vi "PT DIM info service.vi"(1 "serviceName":string, 3 "timeout [ms]":u32=10000, 5 "error in (no error)":errorcluster) -> (14 "serviceID":u32, 15 "data":i8[](array[numeric]), 16 "typeDescriptor":string, 17 "timed out?":bool, 19 "error out":errorcluster)   [LabVIEW 2014, in "PTUtils.lvlib"]
uses:
  PTUtils.lvlib
  CSlibraries-extern/DimLVEvent/LVDimInterface/LVDimInterface.dim service type.ctl
  CSlibraries-extern/DimLVEvent/LVDimInterface/LVDimInterface.dic_info_service_notifier.vi
  CSlibraries-extern/DimLVEvent/LVDimInterface/LVDimInterface.lvlib
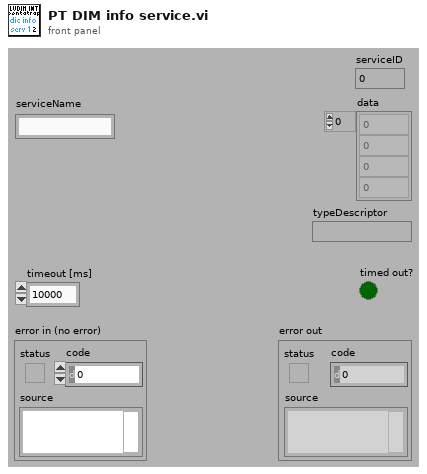
[diagram p1: front panel]
types:
  T1 = typedef "LVDimInterface.lvlib/LVDimInterface.dim service type.ctl" = u16
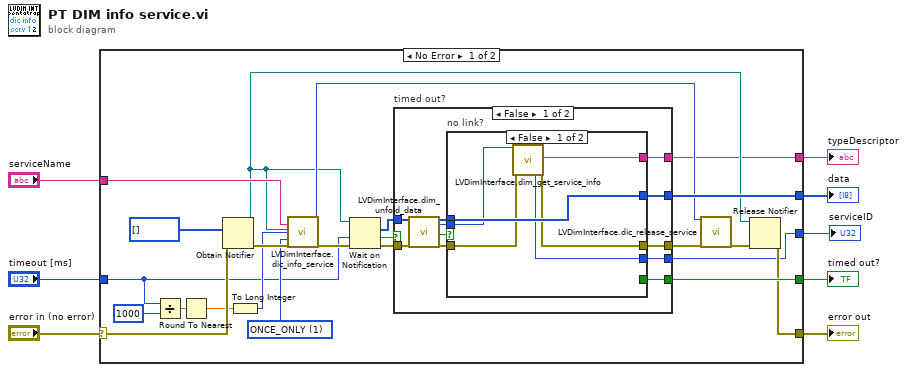
[diagram p0: block diagram]
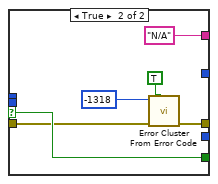
[diagram p2: hidden frame]
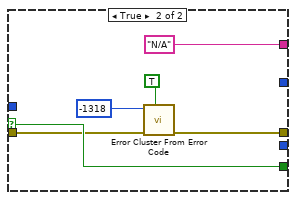
[diagram p3: hidden frame]
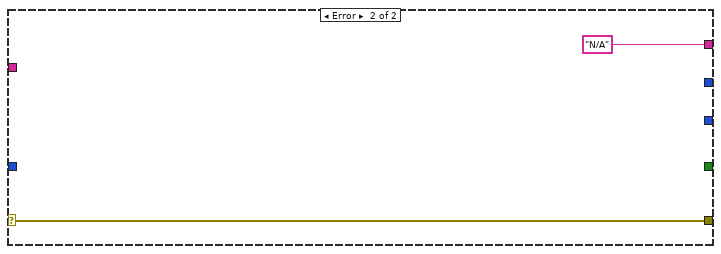
[diagram p4: hidden frame]
diagram:
  n1 = case shown="No Error" "error in (no error)" {
    selector: "error in (no error)" -> [w30 w62]
    tunnel: [w11 w62] -> w7
    tunnel: "serviceName" -> [w22 _]
    tunnel: "timeout [ms]" -> [w16 _]
    tunnel: [w23 _] -> w4
    tunnel: [w21 _] -> w3
    tunnel: [w10 "N/A" ("typeDescriptor")] -> w2
    tunnel: [w9 _] -> w1
    frame No Error {
      w28 = T1 1 items=["ONCE_ONLY"=1, "TIMED"=2, "MONITORED"=4] ("serviceType")
      n2 = Divide(x=w16, y=1000) -> (x/y=w19:dbl)
      n3 = Round To Nearest(number=w19) -> (nearest integer value=w18:dbl)
      n4 = Obtain Notifier(notification data type=i8[] [], error in (no error)=w30) -> (notifier out=w12:refnum<notifier>, error out=w29:errorcluster)  [unwired: 2 in, 1 out]
      n5 = To Long Integer(number=w18) -> (32bit integer=w17:i32)
      n6 = call-poly "LVDimInterface.dic_info_service.vi"("serviceName"=w22, "notifierRef"=w12, "timeout [s]"=w17, "serviceType"=w28, "error in (no error)"=w29) -> ("callBackID"=w14:i32, "error out"=w27:errorcluster)  [unwired: 13 in]
      n7 = Wait on Notification(notifier=w12, timeout in ms (-1)=w16, error in (no error)=w27) -> (notification=w24:i8[], timed out?=w26:bool, error out=w25:errorcluster)  [unwired: 1 in, 1 out]
      n8 = case "timed out?" shown="False" w26 {
        selector: w26 -> [_ w60]
        tunnel: w25 -> [w42 w58]
        tunnel: w24 -> [w41 _]
        tunnel: [w38 _] -> w23
        tunnel: [w37 w60] -> w21
        tunnel: [w36 w57] -> w15
        tunnel: [w34 "N/A" ("typeDescriptor")] -> w10
        tunnel: [w32 _] -> w9
        frame False {
          n9 = call "LVDimInterface.dim_unfold_data.vi"("rawData"=w41, "error in (no error)"=w42) -> ("data"=w39:i8[], "callBackID"=w33:i32, "no link"=w40:bool, "error out"=w35:errorcluster)  [unwired: 14 in]
          n10 = case "no link?" shown="False" w40 {
            selector: w40 -> [_ w54]
            tunnel: [w48 _] -> w38
            tunnel: w39 -> [w48 _]
            tunnel: [_ w54] -> w37
            tunnel: [w44 w51] -> w36
            tunnel: w35 -> [w45 w52]
            tunnel: [w46 "N/A" ("typeDescriptor")] -> w34
            tunnel: w33 -> [w47 _]
            tunnel: [w43 _] -> w32
            frame False {
              n11 = call "LVDimInterface.dim_get_service_info.vi"("callBackID"=w47, "error in (no error)"=w45) -> ("serviceID"=w43:u32, "typeDescriptor"=w46:string, "error out"=w44:errorcluster)  [unwired: 8 in, 7 out]
            }
            frame True {
              n12 = call <vilib>:"Error Cluster From Error Code.vi"("show call chain? (False)"=TRUE ("status"), "error in (no error)"=w52, "error code (0)"=-1318 ("code")) -> ("error out"=w51:errorcluster)  [unwired: 6 in]
            }
          }
        }
        frame True {
          n13 = call <vilib>:"Error Cluster From Error Code.vi"("show call chain? (False)"=TRUE ("status"), "error in (no error)"=w58, "error code (0)"=-1318 ("code")) -> ("error out"=w57:errorcluster)  [unwired: 6 in]
        }
      }
      n14 = call "LVDimInterface.dic_release_service.vi"("callBackID"=w14, "error in (no error)"=w15) -> ("error out"=w13:errorcluster)  [unwired: 17 in]
      n15 = Release Notifier(notifier=w12, error in (no error)=w13) -> (error out=w11:errorcluster)  [unwired: 1 in, 2 out]
    }
    frame Error {
    }
  }
  "error out" <- w7
  "data" <- w4
  "timed out?" <- w3
  "typeDescriptor" <- w2
  "serviceID" <- w1
